vi "Save PNG Image of Front Panel.vi"(8 "error in (no error)":errorcluster, 10 "VI Path":path, 11 "File Path In":path) -> (0 "error out":errorcluster, 3 "File Path Out":path)   [LabVIEW 2012]
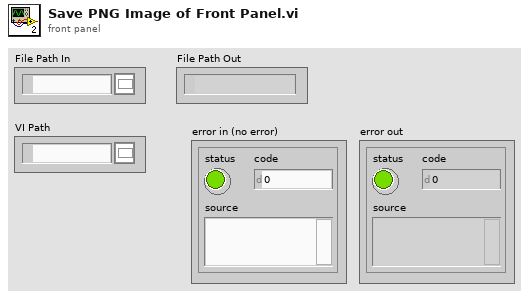
[diagram p1: front panel]
types:
  T1 = typedef "imagedata.ctl" = cluster{"image type":i32, "image depth":i32, "image":u8[], "mask":u8[], "colors":u32[], "Rectangle":cluster{"left":i16, "top":i16, "right":i16, "bottom":i16}}
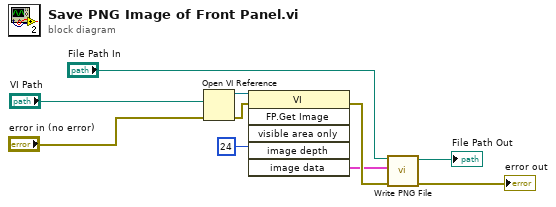
[diagram p0: block diagram]
diagram:
  n1 = Open VI Reference(vi path="VI Path", error in (no error)="error in (no error)") -> (vi reference=w2:refnum<vi>, error out=w7:errorcluster)  [unwired: 4 in]
  n2 = invoke class="VI" method="FP.Get Image"(reference=w2, error in=w7, "image depth"=24 ("Image Depth")) -> (error out=w8:errorcluster, "image data"=w3:T1)  [unwired: 3 in, 4 out]
  n3 = call <vilib>:"Write PNG File.vi"("error in (no error)"=w8, "image data"=w3, "path to PNG file"="File Path In") -> ("error out"=→"error out":errorcluster, "path"=→"File Path Out":path)  [unwired: 7 in]
